vi "fpga_Previous Integration.vi"(6 "instantaneous reset after tripping? (F)":bool, 7 "integrate?":bool, 8 "input valid":bool=TRUE, 10 "channel index":u8, 11 "dt/T":fxp<+/-,32,1>) -> (0 "output valid":bool, 2 "integrated value":fxp<+,32,0>, 3 "trip?":bool)   [LabVIEW 2012, in "NI_EP_Protection_FPGA.lvlib"]
uses:
  <vilib>/addons/Electrical Power/Protection/NI_EP_Protection_FPGA.lvlib
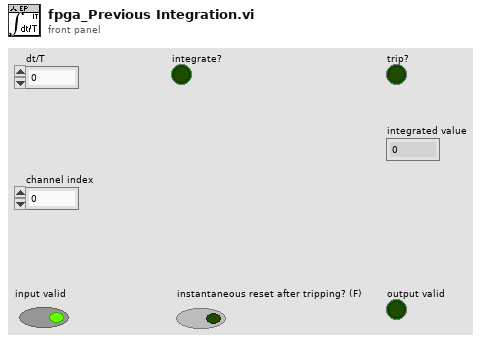
[diagram p1: front panel]
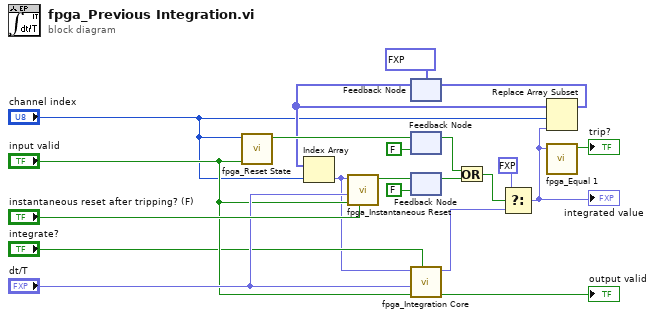
[diagram p0: block diagram]
diagram:
  n1 = call <vilib>:"fpga_Reset State.vi"("input valid"="input valid", "channel index"="channel index") -> ("reset?"=w16:bool)  [unwired: 9 in]
  n2 = feedback #1(fxp<+,32,0>[] [0.0, 0.0, 0.0, 0.0, 0.0, 0.0, 0.0, 0.0, 0.0, 0.0, 0.0, 0.0, 0.0, 0.0, 0.0, 0.0]) -> (w3:fxp<+,32,0>[])
  n3 = Index Array(array=w3, index="channel index") -> (element=w2:fxp<+,32,0>)
  n4 = call <vilib>:"fpga_Instantaneous Reset.vi"("instantaneous reset after tripping? (F)"="instantaneous reset after tripping? (F)", "input valid"="input valid", "dt/T"="dt/T", "previous integrated value"=w2) -> ("instantaneous reset?"=w11:bool)  [unwired: 7 in]
  n5 = feedback #2(FALSE) -> (w15:bool)
  n6 = feedback-in #2(w16) -> ()
  n7 = feedback #3(FALSE) -> (w10:bool)
  n8 = feedback-in #3(w11) -> ()
  n9 = call <vilib>:"fpga_Integration Core.vi"("integrate?"="integrate?", "input valid"="input valid", "dt/T"="dt/T", "previous integrated value"=w2) -> ("output valid"=→"output valid":bool, "integrated value out"=w8:fxp<+,32,0>)  [unwired: 6 in]
  n10 = Or(x=w15, y=w10) -> (x .or. y?=w19:bool)
  n11 = Select(t=fxp<+,32,0> 0.0 ("f"), s=w19, f=w8) -> (s? t:f=w5:fxp<+,32,0>)
  "integrated value" <- w5
  n12 = Replace Array Subset(array=w3, new element=w5, index="channel index") -> (w20:fxp<+,32,0>[])
  n13 = feedback-in #1(w20) -> ()
  n14 = call <vilib>:"fpga_Equal 1.vi"("data in 32.0"=w5) -> ("=1?"=→"trip?":bool)  [unwired: 10 in]
